vi "CRYSet Channel Name Dialog Front Panel.vi"(11 "Vi Ref":refnum<vi>) -> ()   [LabVIEW 2013]
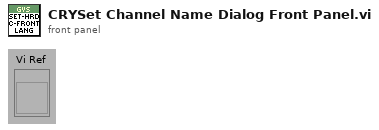
[diagram p1: front panel]
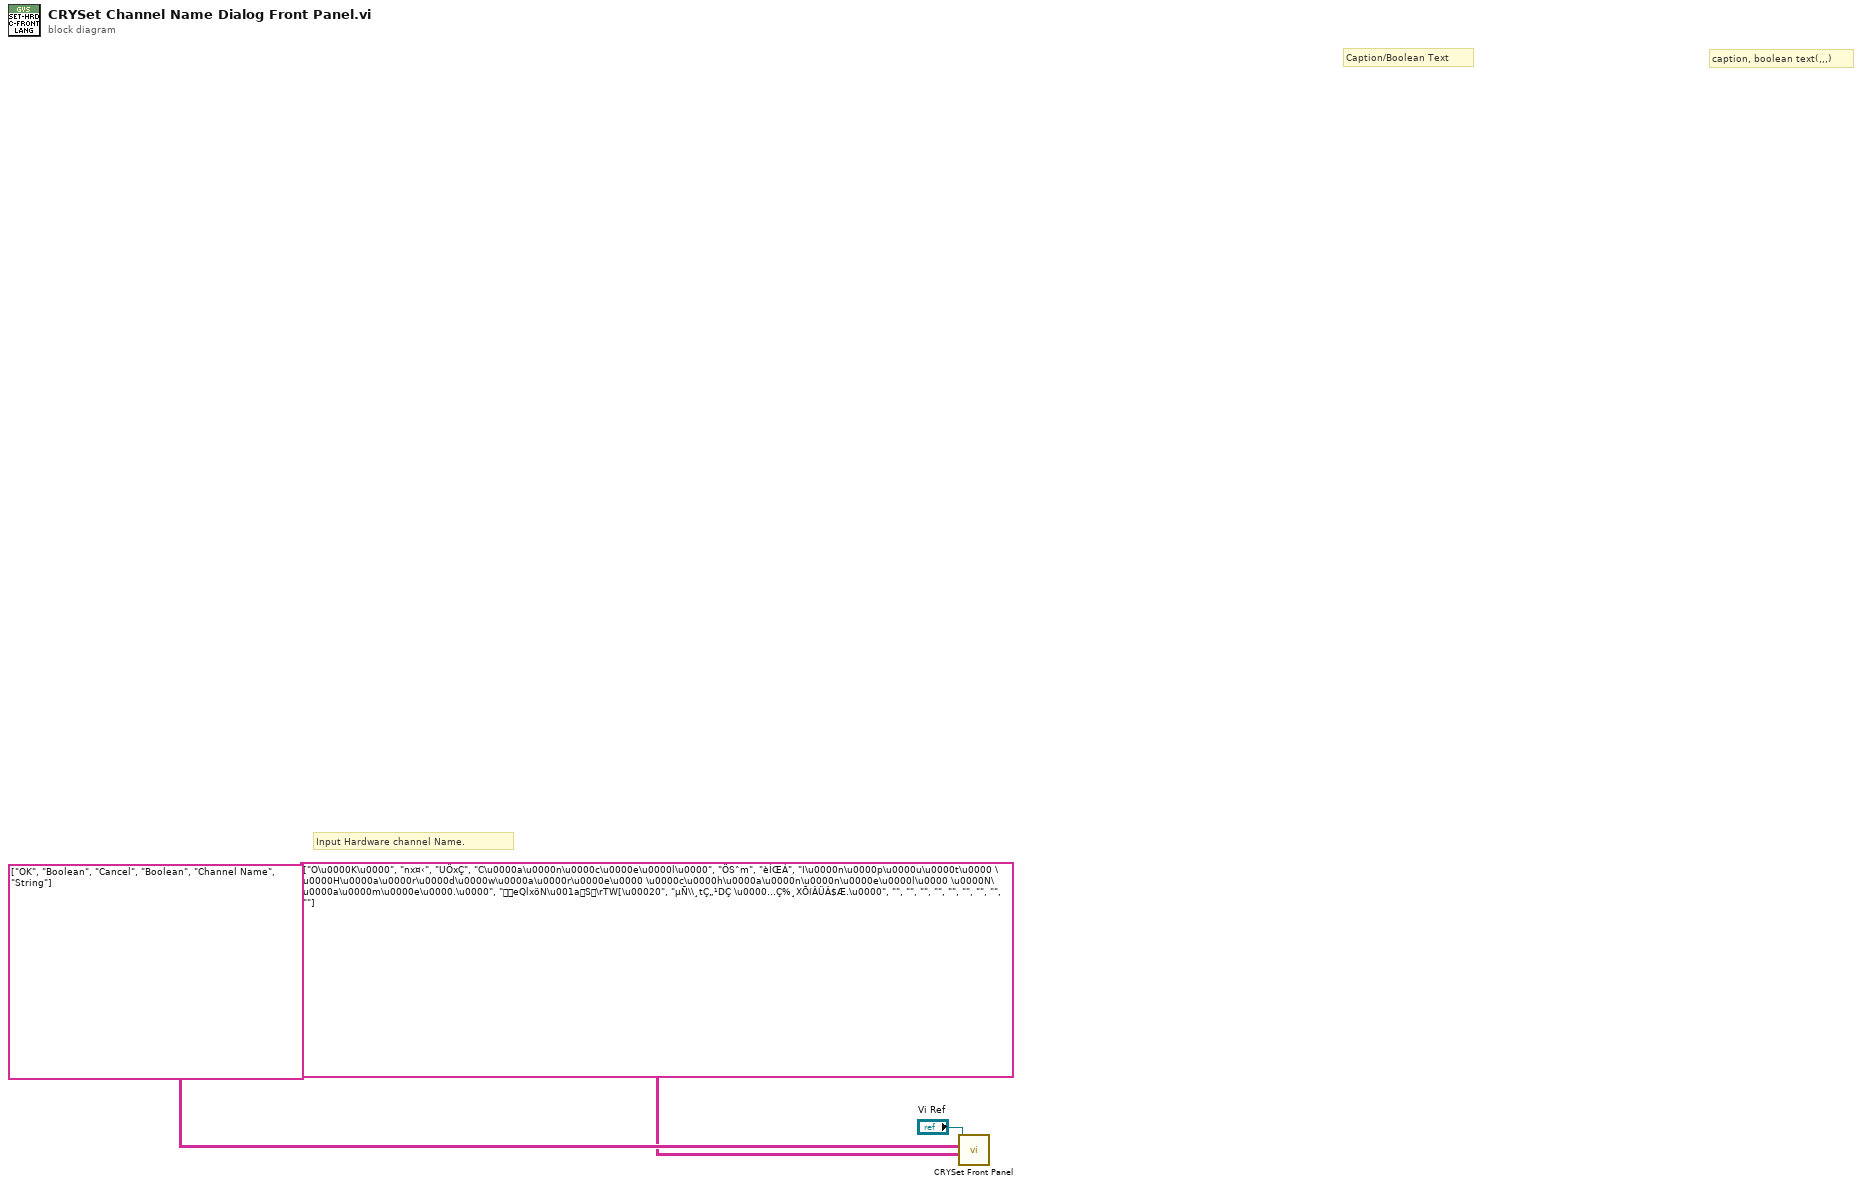
[diagram p0: block diagram]
diagram:
  # "Input Hardware channel Name."
  # "caption, boolean text(,,,)"
  # "Caption/Boolean Text"
  n1 = call "CRYSet Front Panel.vi"("Caption(Boolean Text)"=string[][] [["O\u0000K\u0000", "nx¤‹", "UÖxÇ"], ["C\u0000a\u0000n\u0000c\u0000e\u0000l\u0000", "ÖSˆm", "èÍŒÁ"], ["I\u0000n\u0000p\u0000u\u0000t\u0000 \u0000H\u0000a\u0000r\u0000d\u0000w\u0000a\u0000r\u0000e\u0000 \u0000c\u0000h\u0000a\u0000n\u0000n\u0000e\u0000l\u0000 \u0000N\u0000a\u0000m\u0000e\u0000.\u0000", "eQlxöN\u001aS\rTW[\u00020", "µÑ\\¸tÇ„¹DÇ \u0000…Ç%¸XÕíÂÜÂ$Æ.\u0000"], ["", "", ""], ["", "", ""], ["", "", ""]], "Control ID and Type(Label Name, Type)"=string[][] [["OK", "Boolean"], ["Cancel", "Boolean"], ["Channel Name", "String"]], "Vi Ref"="Vi Ref") -> ()  [unwired: 9 in]
